vi "get fpga resource ref from channels.vi"(1 "channel":refnum<class "TBM channel.lvclass">, 3 "bitfile ref in":refnum<k20>, 5 "error in (no error)":errorcluster) -> (15 "fpga res type":T1, 19 "error out":errorcluster)   [LabVIEW 2015, in "io runtime.lvclass"]
uses:
  <vilib>/NI/Tag Bus Module Framework/channel/TBM channel.lvclass
  configuration/fpga resource supported data types.ctl
  fpga channel/fpga channel.lvclass
  <vilib>/NI/Tag Bus/tag/tag descriptor.lvclass/tag descriptor.ctl
  fpga channel/fpga channel.lvclass/fpga channel.ctl
  FXP I_20_5.ctl
  FXP I_24_5.ctl
  FXP I_24_10.ctl
  <vilib>/NI/LVFPGA Adv Session Resources/OpenByNameSubVI.vi
  <vilib>/NI/Tag Bus/tag/read tag name.vi
  fpga channel/Read FXP type.vi
  <vilib>/NI/Tag Bus/tag/read data type.vi
  <vilib>/rvi/interface/common/dynamic/niFpgaEscapeDelimiterAndNull.vi
  <vilib>/Utility/error.llb/Error Cluster From Error Code.vi
  <vilib>/NI/LVFPGA Adv Session Resources/OpenByName.xnode
  <vilib>/NI/LVFPGA Adv Session Resources/LVFPGAAdvSessionResources.lvlib
  configuration/io configuration.lvclass
  io runtime.lvclass
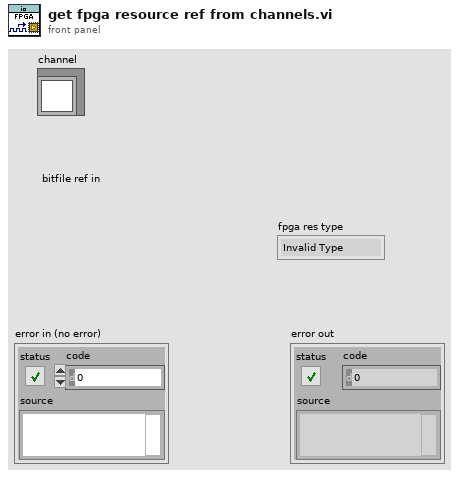
[diagram p1: front panel]
types:
  T1 = typedef "io configuration.lvclass/fpga resource supported data types.ctl" = enum16{"Invalid Type", "Single", "I64", "I32", "I16", "I8", "U64", "U32", "U16", "U8", "Boolean", "FXP I,20,5", "FXP I,24,5", "FXP I,24,10", "Fifo 1023,I16"}
  T2 = cluster{"Name":string, "Depth":u32, "Write? (Deprecated:Use Implementation)":bool, "Physical Channel":u32, "Base Address":u32, "Data Width":u32, "Data Type":enum32{"Boolean", "I8", "I16", "I32", "I64", "U8", "U16", "U32", "U64", "FXP", "CustomControl", "SGL"}, "FXP Properties":variant, "Write Window Address":u32, "Implementation":enum16{"niFpgaTargetToHost", "niFpgaHostToTarget", "niFpgaPeerToPeerWriter", "niFpgaPeerToPeerReader", "niCoreTargetToHost", "niCoreHostToTarget"}, "Control Set":u32}[]
  T3 = cluster{"Name":string, "type":variant, "indicator?":bool}[]
  T4 = typedef "LVFixedPointRepBitsTypeDef.ctl" = cluster{"Signed":bool, "Word Length":u32, "Integer Word Length":i32}
  T5 = typedef "io runtime.lvclass/FXP I_20_5.ctl" = refnum<k20>
  T6 = typedef "io runtime.lvclass/FXP I_24_5.ctl" = refnum<k20>
  T7 = typedef "io runtime.lvclass/FXP I_24_10.ctl" = refnum<k20>
  T8 = typedef "tag bus.lvlib/tag descriptor.lvclass/Data Type.ctl" = enum16{"Double", "Single", "I64", "I32", "I16", "I8", "U64", "U32", "U16", "U8", "Boolean", "String", "Array of Double", "Array of Single", "Array of I64", "Array of I32", "Array of I16", "Array of I8", "Array of U64", "Array of U32", "Array of U16", "Array of U8", "Array of Boolean", "Array of String"}
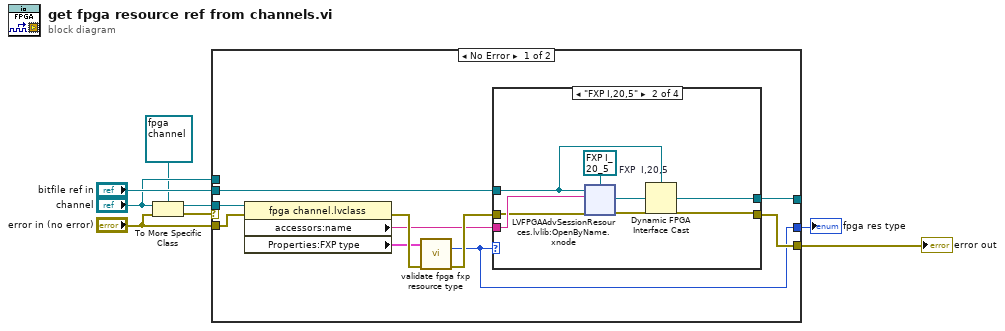
[diagram p0: block diagram]
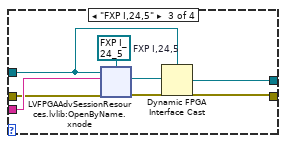
[diagram p3: hidden frame]
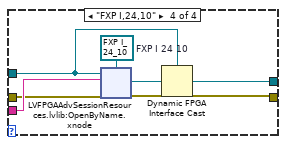
[diagram p4: hidden frame]
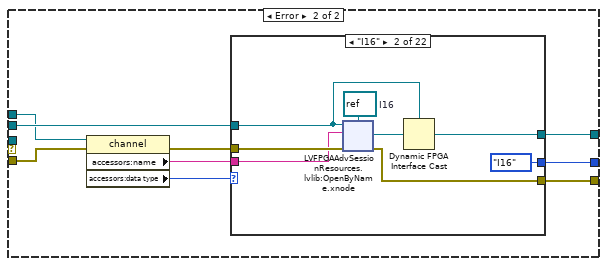
[diagram p5: hidden frame]
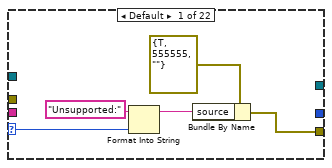
[diagram p6: hidden frame]
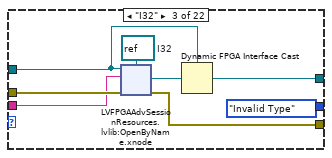
[diagram p7: hidden frame]
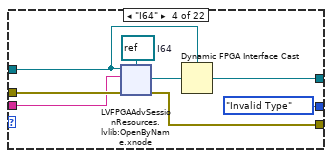
[diagram p8: hidden frame]
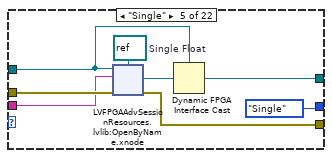
[diagram p9: hidden frame]
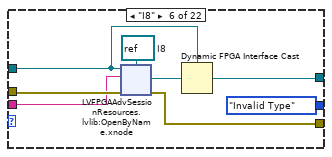
[diagram p10: hidden frame]
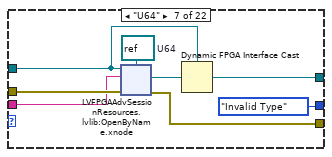
[diagram p11: hidden frame]
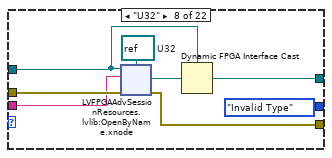
[diagram p12: hidden frame]
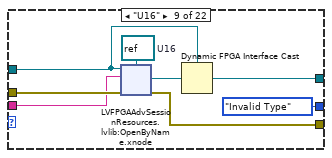
[diagram p13: hidden frame]
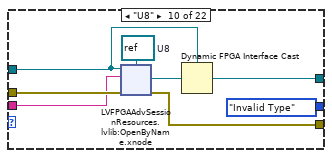
[diagram p14: hidden frame]
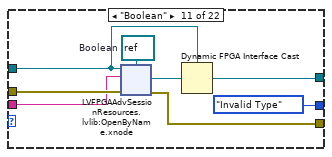
[diagram p15: hidden frame]
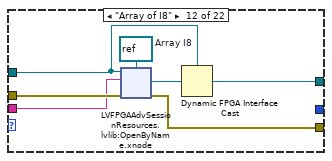
[diagram p16: hidden frame]
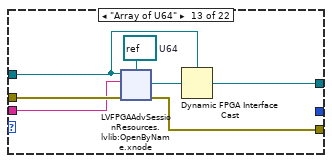
[diagram p17: hidden frame]
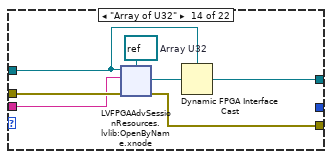
[diagram p18: hidden frame]
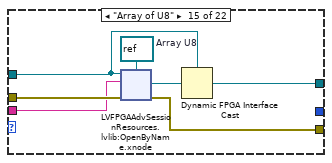
[diagram p19: hidden frame]
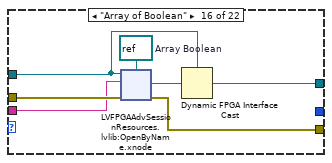
[diagram p20: hidden frame]
diagram:
  n1 = To More Specific Class(target class=refnum<class "fpga channel.lvclass"> refnum ("Fxp Channel.lvclass"), reference="channel", error in="error in (no error)") -> (specific class reference=w7:refnum<class "fpga channel.lvclass">, error out=w8:errorcluster)
  n2 = case shown="No Error" w8 {
    tunnel: w7 -> [w16 _]
    tunnel: "bitfile ref in" -> [w15 w83]
    tunnel: [w12 w84] -> w2
    tunnel: [w14 w88] -> _
    tunnel: [w10 w80] -> w5
    tunnel: "channel" -> [_ w82]
    tunnel: "error in (no error)" -> [w9 w81]
    frame No Error {
      n3 = property class="fpga channel.lvclass"(reference=w16, error in=w9) -> (error out=w18:errorcluster, "accessors:name"=w13:string, "Properties:FXP type"=w11:T4)  [unwired: 1 out]
      n4 = call "validate fpga fxp resource type.vi"("FXP Representation"=w11, "error in (no error)"=w18) -> ("fpga res type"=w10:T1, "error out"=w17:errorcluster)  [unwired: 11 in, 1 out]
      n5 = case shown="\"FXP I,20,5\"" w10 {
        tunnel: w15 -> [_ w21 w46 w65]
        tunnel: [_ w25 w45 w64] -> w14
        tunnel: w13 -> [_ w24 w44 w63]
        tunnel: w17 -> [w19 w23 w43 w62]
        tunnel: [w19 w22 w42 w61] -> w12
        frame "Invalid Type", Default {
        }
        frame "FXP I,20,5" {
          w20 = T5 refnum  # FXP  I,20,5
          n6 = xnode "LVFPGAAdvSessionResources.lvlib:OpenByName.xnode"("FPGA VI Reference in"=w21, "Resource name in"=w24, "Single resource reference type in"=w20, "Error in"=w23) -> ("Single resource reference out"=w26:T5, "Error out"=w22:errorcluster)  [unwired: 1 out]
          n7 = Dynamic FPGA Interface Cast(Session In=w21, Type=w26) -> (Session Out=w25:refnum<k20>)
        }
        frame "FXP I,24,5" {
          w40 = T6 refnum  # FXP I,24,5
          n8 = xnode "LVFPGAAdvSessionResources.lvlib:OpenByName.xnode"("FPGA VI Reference in"=w46, "Resource name in"=w44, "Single resource reference type in"=w40, "Error in"=w43) -> ("Single resource reference out"=w41:T6, "Error out"=w42:errorcluster)  [unwired: 1 out]
          n9 = Dynamic FPGA Interface Cast(Session In=w46, Type=w41) -> (Session Out=w45:refnum<k20>)
        }
        frame "FXP I,24,10" {
          w60 = T7 refnum  # FXP I 24 10
          n10 = xnode "LVFPGAAdvSessionResources.lvlib:OpenByName.xnode"("FPGA VI Reference in"=w65, "Resource name in"=w63, "Single resource reference type in"=w60, "Error in"=w62) -> ("Single resource reference out"=w66:T7, "Error out"=w61:errorcluster)  [unwired: 1 out]
          n11 = Dynamic FPGA Interface Cast(Session In=w65, Type=w66) -> (Session Out=w64:refnum<k20>)
        }
      }
    }
    frame Error {
      n12 = property class="channel"(reference=w82, error in=w81) -> (error out=w87:errorcluster, "accessors:name"=w85:string, "accessors:data type"=w86:T8)  [unwired: 1 out]
      n13 = case shown="\"I16\"" w86 {
        selector: w86 -> [w91 _ _ _ _ _ _ _ _ _ _ _ _ _ _ _ _ _ _ _ _ _]
        tunnel: w87 -> [_ w101 w122 w143 w164 w185 w206 w227 w248 w269 w290 w310 w330 w350 w370 w390 w410 w430 w450 w470 w490 w510]
        tunnel: [w93 w100 w121 w142 w163 w184 w205 w226 w247 w268 w289 w309 w329 w349 w369 w389 w409 w424 w449 w469 w489 w509] -> w84
        tunnel: w83 -> [_ w98 w119 w140 w161 w182 w203 w224 w245 w266 w287 w307 w327 w347 w367 w387 w406 w427 w446 w466 w486 w506]
        tunnel: w85 -> [_ w99 w120 w141 w162 w183 w204 w225 w246 w267 w288 w308 w328 w348 w368 w388 w408 w429 w448 w468 w488 w508]
        tunnel: [_ w97 w118 w139 w160 w181 w202 w223 w244 w265 w286 w306 w326 w346 w366 w386 w405 w426 w445 w465 w485 w505] -> w88
        tunnel: [_ fpga_resource_supported_data_types."I16" ("fpga res type") fpga_resource_supported_data_types."Invalid Type" ("fpga res type") fpga_resource_supported_data_types."Invalid Type" ("fpga res type") fpga_resource_supported_data_types."Single" ("fpga res type") fpga_resource_supported_data_types."Invalid Type" ("fpga res type") fpga_resource_supported_data_types."Invalid Type" ("fpga res type") fpga_resource_supported_data_types."Invalid Type" ("fpga res type") fpga_resource_supported_data_types."Invalid Type" ("fpga res type") fpga_resource_supported_data_types."Invalid Type" ("fpga res type") fpga_resource_supported_data_types."Invalid Type" ("fpga res type") _ _ _ _ _ _ _ _ _ _ _] -> w80
        frame Default {
          n14 = Format Into String(initial string="Unsupported:" ("source"), w91) -> (resulting string=w89:string)  [unwired: 2 in, 1 out]
          n15 = Bundle By Name(cluster=errorcluster {"status"=TRUE, "code"=555555, "source"=""} ("Error out"), "source"=w89) -> (w93:errorcluster)
        }
        frame "I16" {
          w96 = refnum<k20> refnum  # I16
          n16 = xnode "LVFPGAAdvSessionResources.lvlib:OpenByName.xnode"("FPGA VI Reference in"=w98, "Resource name in"=w99, "Single resource reference type in"=w96, "Error in"=w101) -> ("Single resource reference out"=w95:refnum<k20>, "Error out"=w100:errorcluster)  [unwired: 1 out]
          n17 = Dynamic FPGA Interface Cast(Session In=w98, Type=w95) -> (Session Out=w97:refnum<k20>)
        }
        frame "I32" {
          w117 = refnum<k20> refnum  # I32
          n18 = xnode "LVFPGAAdvSessionResources.lvlib:OpenByName.xnode"("FPGA VI Reference in"=w119, "Resource name in"=w120, "Single resource reference type in"=w117, "Error in"=w122) -> ("Single resource reference out"=w116:refnum<k20>, "Error out"=w121:errorcluster)  [unwired: 1 out]
          n19 = Dynamic FPGA Interface Cast(Session In=w119, Type=w116) -> (Session Out=w118:refnum<k20>)
        }
        frame "I64" {
          w138 = refnum<k20> refnum  # I64
          n20 = xnode "LVFPGAAdvSessionResources.lvlib:OpenByName.xnode"("FPGA VI Reference in"=w140, "Resource name in"=w141, "Single resource reference type in"=w138, "Error in"=w143) -> ("Single resource reference out"=w137:refnum<k20>, "Error out"=w142:errorcluster)  [unwired: 1 out]
          n21 = Dynamic FPGA Interface Cast(Session In=w140, Type=w137) -> (Session Out=w139:refnum<k20>)
        }
        frame "Single" {
          w159 = refnum<k20> refnum  # Single Float
          n22 = xnode "LVFPGAAdvSessionResources.lvlib:OpenByName.xnode"("FPGA VI Reference in"=w161, "Resource name in"=w162, "Single resource reference type in"=w159, "Error in"=w164) -> ("Single resource reference out"=w158:refnum<k20>, "Error out"=w163:errorcluster)  [unwired: 1 out]
          n23 = Dynamic FPGA Interface Cast(Session In=w161, Type=w158) -> (Session Out=w160:refnum<k20>)
        }
        frame "I8" {
          w180 = refnum<k20> refnum  # I8
          n24 = xnode "LVFPGAAdvSessionResources.lvlib:OpenByName.xnode"("FPGA VI Reference in"=w182, "Resource name in"=w183, "Single resource reference type in"=w180, "Error in"=w185) -> ("Single resource reference out"=w179:refnum<k20>, "Error out"=w184:errorcluster)  [unwired: 1 out]
          n25 = Dynamic FPGA Interface Cast(Session In=w182, Type=w179) -> (Session Out=w181:refnum<k20>)
        }
        frame "U64" {
          w201 = refnum<k20> refnum  # U64
          n26 = xnode "LVFPGAAdvSessionResources.lvlib:OpenByName.xnode"("FPGA VI Reference in"=w203, "Resource name in"=w204, "Single resource reference type in"=w201, "Error in"=w206) -> ("Single resource reference out"=w200:refnum<k20>, "Error out"=w205:errorcluster)  [unwired: 1 out]
          n27 = Dynamic FPGA Interface Cast(Session In=w203, Type=w200) -> (Session Out=w202:refnum<k20>)
        }
        frame "U32" {
          w222 = refnum<k20> refnum  # U32
          n28 = xnode "LVFPGAAdvSessionResources.lvlib:OpenByName.xnode"("FPGA VI Reference in"=w224, "Resource name in"=w225, "Single resource reference type in"=w222, "Error in"=w227) -> ("Single resource reference out"=w221:refnum<k20>, "Error out"=w226:errorcluster)  [unwired: 1 out]
          n29 = Dynamic FPGA Interface Cast(Session In=w224, Type=w221) -> (Session Out=w223:refnum<k20>)
        }
        frame "U16" {
          w243 = refnum<k20> refnum  # U16
          n30 = xnode "LVFPGAAdvSessionResources.lvlib:OpenByName.xnode"("FPGA VI Reference in"=w245, "Resource name in"=w246, "Single resource reference type in"=w243, "Error in"=w248) -> ("Single resource reference out"=w242:refnum<k20>, "Error out"=w247:errorcluster)  [unwired: 1 out]
          n31 = Dynamic FPGA Interface Cast(Session In=w245, Type=w242) -> (Session Out=w244:refnum<k20>)
        }
        frame "U8" {
          w264 = refnum<k20> refnum  # U8
          n32 = xnode "LVFPGAAdvSessionResources.lvlib:OpenByName.xnode"("FPGA VI Reference in"=w266, "Resource name in"=w267, "Single resource reference type in"=w264, "Error in"=w269) -> ("Single resource reference out"=w263:refnum<k20>, "Error out"=w268:errorcluster)  [unwired: 1 out]
          n33 = Dynamic FPGA Interface Cast(Session In=w266, Type=w263) -> (Session Out=w265:refnum<k20>)
        }
        frame "Boolean" {
          w285 = refnum<k20> refnum  # Boolean
          n34 = xnode "LVFPGAAdvSessionResources.lvlib:OpenByName.xnode"("FPGA VI Reference in"=w287, "Resource name in"=w288, "Single resource reference type in"=w285, "Error in"=w290) -> ("Single resource reference out"=w284:refnum<k20>, "Error out"=w289:errorcluster)  [unwired: 1 out]
          n35 = Dynamic FPGA Interface Cast(Session In=w287, Type=w284) -> (Session Out=w286:refnum<k20>)
        }
        frame "Array of I8" {
          w304 = refnum<k20> refnum  # Array I8
          n36 = xnode "LVFPGAAdvSessionResources.lvlib:OpenByName.xnode"("FPGA VI Reference in"=w307, "Resource name in"=w308, "Single resource reference type in"=w304, "Error in"=w310) -> ("Single resource reference out"=w305:refnum<k20>, "Error out"=w309:errorcluster)  [unwired: 1 out]
          n37 = Dynamic FPGA Interface Cast(Session In=w307, Type=w305) -> (Session Out=w306:refnum<k20>)
        }
        frame "Array of U64" {
          w324 = refnum<k20> refnum  # U64
          n38 = xnode "LVFPGAAdvSessionResources.lvlib:OpenByName.xnode"("FPGA VI Reference in"=w327, "Resource name in"=w328, "Single resource reference type in"=w324, "Error in"=w330) -> ("Single resource reference out"=w325:refnum<k20>, "Error out"=w329:errorcluster)  [unwired: 1 out]
          n39 = Dynamic FPGA Interface Cast(Session In=w327, Type=w325) -> (Session Out=w326:refnum<k20>)
        }
        frame "Array of U32" {
          w344 = refnum<k20> refnum  # Array U32
          n40 = xnode "LVFPGAAdvSessionResources.lvlib:OpenByName.xnode"("FPGA VI Reference in"=w347, "Resource name in"=w348, "Single resource reference type in"=w344, "Error in"=w350) -> ("Single resource reference out"=w345:refnum<k20>, "Error out"=w349:errorcluster)  [unwired: 1 out]
          n41 = Dynamic FPGA Interface Cast(Session In=w347, Type=w345) -> (Session Out=w346:refnum<k20>)
        }
        frame "Array of U8" {
          w364 = refnum<k20> refnum  # Array U8
          n42 = xnode "LVFPGAAdvSessionResources.lvlib:OpenByName.xnode"("FPGA VI Reference in"=w367, "Resource name in"=w368, "Single resource reference type in"=w364, "Error in"=w370) -> ("Single resource reference out"=w365:refnum<k20>, "Error out"=w369:errorcluster)  [unwired: 1 out]
          n43 = Dynamic FPGA Interface Cast(Session In=w367, Type=w365) -> (Session Out=w366:refnum<k20>)
        }
        frame "Array of Boolean" {
          w384 = refnum<k20> refnum  # Array Boolean
          n44 = xnode "LVFPGAAdvSessionResources.lvlib:OpenByName.xnode"("FPGA VI Reference in"=w387, "Resource name in"=w388, "Single resource reference type in"=w384, "Error in"=w390) -> ("Single resource reference out"=w385:refnum<k20>, "Error out"=w389:errorcluster)  [unwired: 1 out]
          n45 = Dynamic FPGA Interface Cast(Session In=w387, Type=w385) -> (Session Out=w386:refnum<k20>)
        }
        frame "Array of Single" {
          w404 = refnum<k20> refnum  # Array Single
          n46 = xnode "LVFPGAAdvSessionResources.lvlib:OpenByName.xnode"("FPGA VI Reference in"=w406, "Resource name in"=w408, "Single resource reference type in"=w404, "Error in"=w410) -> ("Single resource reference out"=w407:refnum<k20>, "Error out"=w409:errorcluster)  [unwired: 1 out]
          n47 = Dynamic FPGA Interface Cast(Session In=w406, Type=w407) -> (Session Out=w405:refnum<k20>)
        }
        frame "Array of Double" {
          w425 = refnum<k20> refnum  # FXP
          n48 = xnode "LVFPGAAdvSessionResources.lvlib:OpenByName.xnode"("FPGA VI Reference in"=w427, "Resource name in"=w429, "Single resource reference type in"=w425, "Error in"=w430) -> ("Single resource reference out"=w428:refnum<k20>, "Error out"=w424:errorcluster)  [unwired: 1 out]
          n49 = Dynamic FPGA Interface Cast(Session In=w427, Type=w428) -> (Session Out=w426:refnum<k20>)
        }
        frame "Array of I64" {
          w444 = refnum<k20> refnum  # Array I64
          n50 = xnode "LVFPGAAdvSessionResources.lvlib:OpenByName.xnode"("FPGA VI Reference in"=w446, "Resource name in"=w448, "Single resource reference type in"=w444, "Error in"=w450) -> ("Single resource reference out"=w447:refnum<k20>, "Error out"=w449:errorcluster)  [unwired: 1 out]
          n51 = Dynamic FPGA Interface Cast(Session In=w446, Type=w447) -> (Session Out=w445:refnum<k20>)
        }
        frame "Array of I32" {
          w464 = refnum<k20> refnum  # Array I32
          n52 = xnode "LVFPGAAdvSessionResources.lvlib:OpenByName.xnode"("FPGA VI Reference in"=w466, "Resource name in"=w468, "Single resource reference type in"=w464, "Error in"=w470) -> ("Single resource reference out"=w467:refnum<k20>, "Error out"=w469:errorcluster)  [unwired: 1 out]
          n53 = Dynamic FPGA Interface Cast(Session In=w466, Type=w467) -> (Session Out=w465:refnum<k20>)
        }
        frame "Array of I16" {
          w484 = refnum<k20> refnum  # Array I16
          n54 = xnode "LVFPGAAdvSessionResources.lvlib:OpenByName.xnode"("FPGA VI Reference in"=w486, "Resource name in"=w488, "Single resource reference type in"=w484, "Error in"=w490) -> ("Single resource reference out"=w487:refnum<k20>, "Error out"=w489:errorcluster)  [unwired: 1 out]
          n55 = Dynamic FPGA Interface Cast(Session In=w486, Type=w487) -> (Session Out=w485:refnum<k20>)
        }
        frame "Array of U16" {
          w504 = refnum<k20> refnum  # Array U16
          n56 = xnode "LVFPGAAdvSessionResources.lvlib:OpenByName.xnode"("FPGA VI Reference in"=w506, "Resource name in"=w508, "Single resource reference type in"=w504, "Error in"=w510) -> ("Single resource reference out"=w507:refnum<k20>, "Error out"=w509:errorcluster)  [unwired: 1 out]
          n57 = Dynamic FPGA Interface Cast(Session In=w506, Type=w507) -> (Session Out=w505:refnum<k20>)
        }
      }
    }
  }
  "error out" <- w2
  "fpga res type" <- w5
